vi "Error Builder.vi"(0 "Error String":string, 1 "is warning? (False)":bool, 11 "Error In":errorcluster) -> (15 "Error Out":errorcluster)   [LabVIEW 2021]
doc: "Builds the custom error based on the input error string and Error In input"
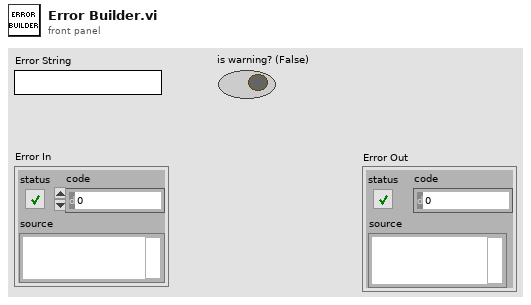
[diagram p1: front panel]
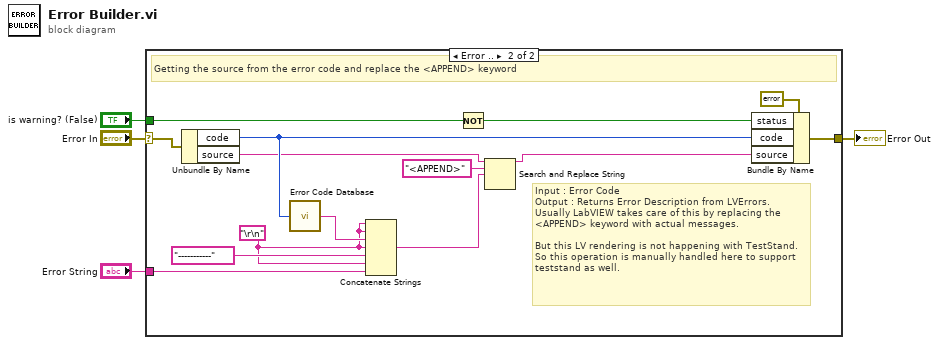
[diagram p0: block diagram]
diagram:
  n1 = case shown="Error .." "Error In" {
    selector: "Error In" -> [w5 w18]
    tunnel: [w5 w12] -> w4
    tunnel: "Error String" -> [_ w17]
    tunnel: "is warning? (False)" -> [_ w15]
    frame No Error {
      # "Skipping the error building operation"
    }
    frame Error {
      w6 = "\r\n" ("End of Line Constant")
      # "Input : Error Code\nOutput : Returns Error Description from LVErrors.\nUsually LabVIEW takes care of this by replacing the <APPEND> keyword with actual messages.\n\nBut this LV rendering is not happening with TestStand. So this operation is manually handled here to support teststand as well."
      # "Getting the source from the error code and replace the <APPEND> keyword"
      n2 = Unbundle By Name(w18) -> ("code"=w13:i32, "source"=w10:string)
      n3 = call <vilib>:"Error Code Database.vi"("Error Code"=w13) -> ("Error Text"=w7:string)
      n4 = Concatenate Strings(w6, w6, w7, w6, "-----------" ("string"), w6, w17) -> (w9:string)
      n5 = Not(x=w15) -> (.not. x?=w14:bool)
      n6 = Search and Replace String(input string=w10, search string="<APPEND>" ("regular expression"), replace string=w9) -> (result string=w8:string)  [unwired: 5 in, 3 out]
      n7 = Bundle By Name(cluster=errorcluster {"status"=FALSE, "code"=0, "source"=""} ("error out"), "status"=w14, "code"=w13, "source"=w8) -> (w12:errorcluster)
    }
  }
  "Error Out" <- w4
